vi "Host Key Length.vi"(8 "Error In":errorcluster, 11 "Session In":refnum<class "Session.lvclass">) -> (0 "Error Out":errorcluster, 2 "Length":i32, 3 "Sesssion Out":refnum<class "Session.lvclass">)   [LabVIEW 2021, in "Field_RnD_Services_LIBSSH2_Toolkit.lvlib" / "Session.lvclass"]
doc: "Gets the length in bytes (B) of the public host key's binary data."
uses:
  Session.lvclass
  Field_RnD_Services_LIBSSH2_Toolkit.lvlib
  SSH/SSH.lvclass
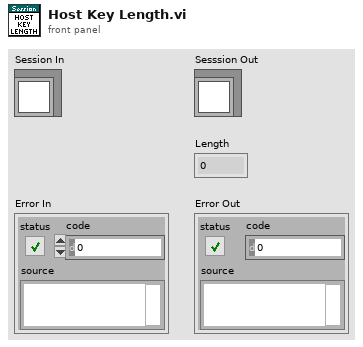
[diagram p1: front panel]
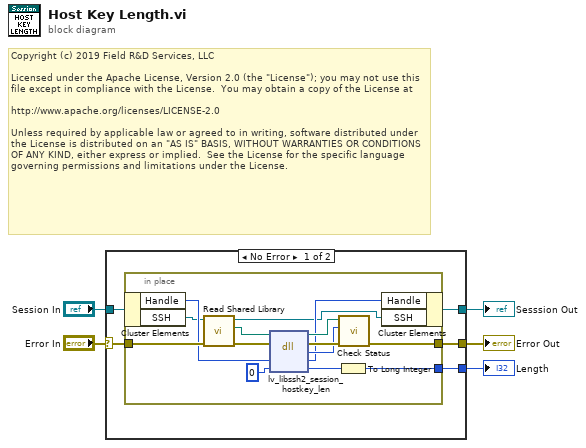
[diagram p0: block diagram]
diagram:
  # "Copyright (c) 2019 Field R&D Services, LLC\n\nLicensed under the Apache License, Version 2.0 (the \"License\"); you may not use this file except in compliance with the License.  You may obtain a copy of the License at\n\nhttp://www.apache.org/licenses/LICENSE-2.0\n\nUnless required by applicable law or agreed to in writing, software distributed under the License is distributed on an \"AS IS\" BASIS, WITHOUT WARRANTIES OR CONDITIONS OF ANY KIND, either express or implied.  See the License for the specific language governing permissions and limitations under the License."
  n1 = case shown="No Error" "Error In" {
    selector: "Error In" -> [w10 w26]
    tunnel: [w7 w26] -> w4
    tunnel: "Session In" -> [w9 w25]
    tunnel: [w8 w25] -> w2
    tunnel: [w6 _] -> w1
    frame No Error {
      n2 = in-place {
        in-place-border: w10 -> [w21]
        in-place-border: [w20] -> w7
        in-place-border: [w18] -> w6
        n3 = in-place-cluster #1(w9) -> ("Handle"=w17:u64, "SSH"=w13:refnum<class "SSH.lvclass">)
        n4 = call "Read Shared Library.vi"("Error In"=w21, "SSH In"=w13) -> ("Error Out"=w14:errorcluster, "libssh2lv Shared Library"=w11:path, "SSH Out"=w12:refnum<class "SSH.lvclass">)  [unwired: 7 in]
        n5 = dll-call lib="D:/Users/cfield/Code/Field R&D Services/SSH/LV-LIBSSH2/LabVIEW/trunk/src/Toolkit/Support/lv-libssh2.*" fn="lv_libssh2_session_hostkey_len"(path in=w11, error in=w14, "handle"=w17, "length"=u64 0) -> (path out=w23:path, error out=w24:errorcluster, "status"=w22:i32, "handle"=w16:u64, "length"=w19:u64)  [unwired: 1 in]
        n6 = To Long Integer(number=w19) -> (32bit integer=w18:i32)
        n7 = call "Check Status.vi"("Error In"=w24, "Status"=w22, "libssh2lv Shared Library In"=w23) -> ("Error Out"=w20:errorcluster)  [unwired: 7 in, 1 out]
        n8 = in-place-cluster #1("Handle"=w16, "SSH"=w12) -> (w8:refnum<class "Session.lvclass">)
      }
    }
    frame Error {
    }
  }
  "Sesssion Out" <- w2
  "Error Out" <- w4
  "Length" <- w1
